vi "GetRange.vi"(8 "error in (no error)":errorcluster, 11 "HAMAMATSU_DCAMAPI in":refnum<class "HAMAMATSU_DCAMAPI.lvclass">) -> (0 "error out":errorcluster, 3 "HAMAMATSU_DCAMAPI out":refnum<class "HAMAMATSU_DCAMAPI.lvclass">)   [LabVIEW 2020, in "HAMAMATSU_DCAMAPI.lvclass"]
uses:
  HAMAMATSU_DCAMAPI.lvclass
  Image Acquisition Class/Camera.lvclass
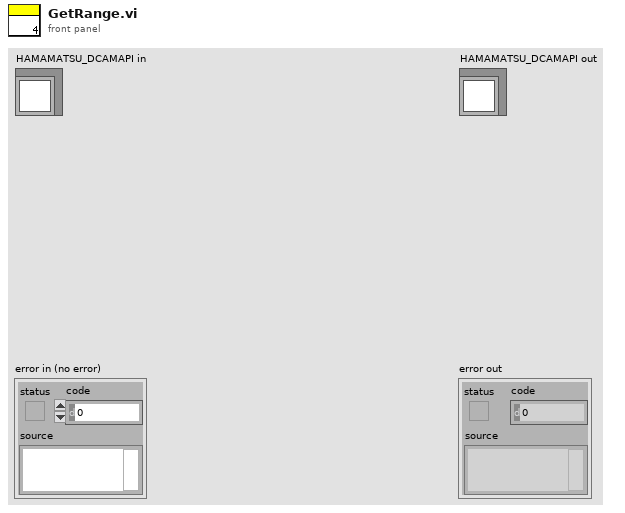
[diagram p1: front panel]
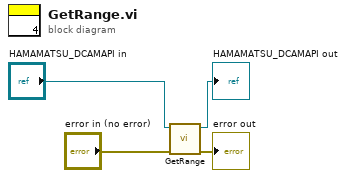
[diagram p0: block diagram]
diagram:
  n1 = call-parent "GetRange.vi"("error in (no error)"="error in (no error)", "Camera in"="HAMAMATSU_DCAMAPI in") -> ("error out"=→"error out":errorcluster, "Camera out"=→"HAMAMATSU_DCAMAPI out":refnum<class "HAMAMATSU_DCAMAPI.lvclass">)  [unwired: 8 in]
